vi "UploadImages.vi"(8 "error in (no error)":errorcluster, 11 "Vision in":refnum<class "Vision.lvclass">) -> (0 "error out":errorcluster, 3 "Vision out":refnum<class "Vision.lvclass">)   [LabVIEW 2019, in "Vision.lvlib" / "Vision.lvclass"]
uses:
  Vision.lvclass
  C:/Program Files/National Instruments/LabVIEW 2019/vi.lib/ActorFramework/Actor/Actor.lvclass
  <vilib>/ActorFramework/Actor/Actor.lvclass/Actor.ctl
  Vision.lvclass/Vision.ctl
  Models/ImagesModel.ctl
  Vision Messages/CapturedImage Msg/CapturedImage Msg.lvclass/CapturedImage Msg.ctl
  <vilib>/ActorFramework/Message Enqueuer/Message Enqueuer.lvclass/Message Enqueuer.ctl
  <vilib>/ActorFramework/Message Enqueuer/Enqueue.vi
  Vision Messages/CapturedImage Msg/CapturedImage Msg.lvclass
  C:/Program Files/National Instruments/LabVIEW 2019/vi.lib/ActorFramework/Message/Message.lvclass
  <vilib>/ActorFramework/Message Priority Queue/Priority Enqueue.vi
  <vilib>/ActorFramework/Message Enqueuer/Message Enqueuer.lvclass
  <vilib>/ActorFramework/Actor/Actor.lvclass
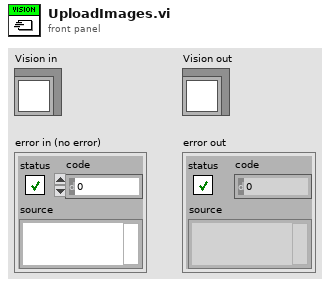
[diagram p1: front panel]
types:
  T1 = typedef "ImagesModel.ctl" = cluster{"guid":string, "images":cluster{"source":string, "rois":string[]}}
  T2 = typedef "IMAQ Image.ctl" = refnum<image>
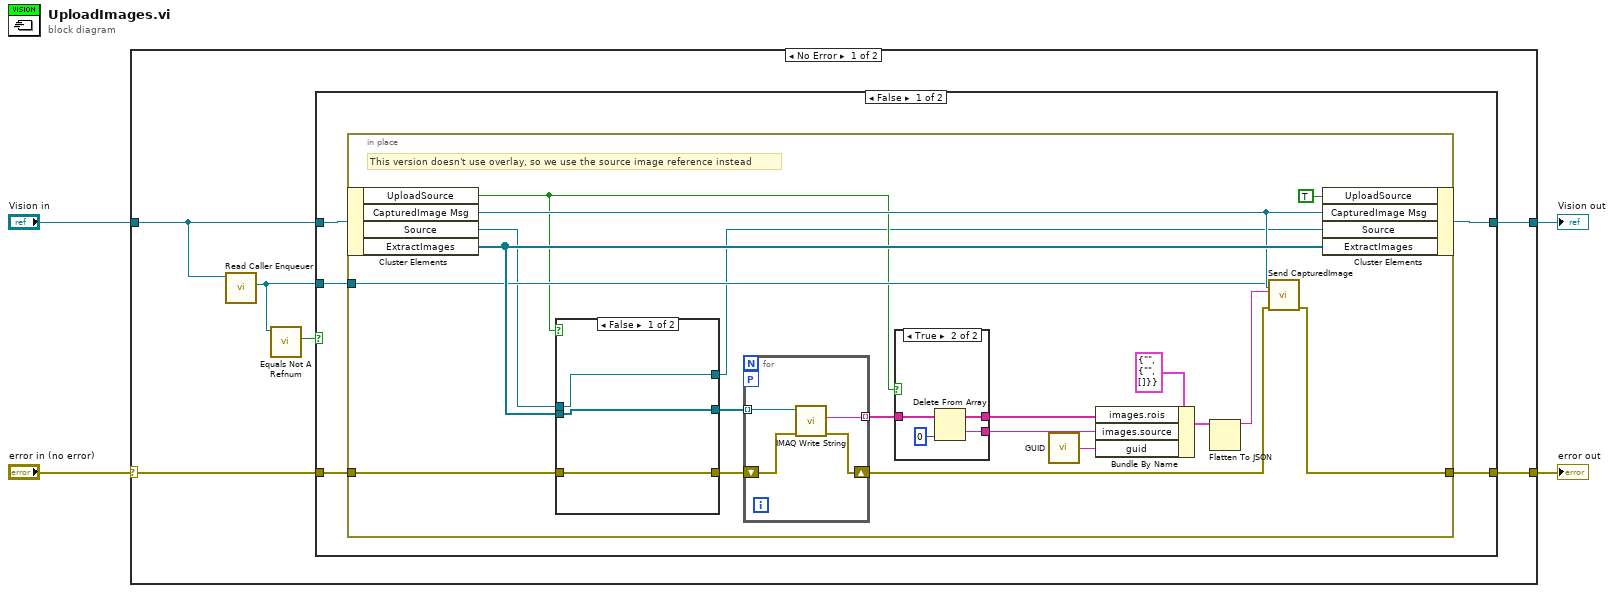
[diagram p0: block diagram]
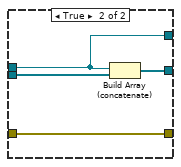
[diagram p2: hidden frame]
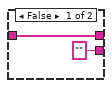
[diagram p3: hidden frame]
diagram:
  n1 = case shown="No Error" "error in (no error)" {
    selector: "error in (no error)" -> [w8 w55]
    tunnel: [w7 w55] -> w3
    tunnel: [w9 w54] -> w1
    tunnel: "Vision in" -> [w10 w54]
    frame No Error {
      n2 = call <vilib>:"Read Caller Enqueuer.vi"("Actor"=w10) -> ("Caller Enqueuer"=w5:refnum<class "Message Enqueuer.lvclass">)  [unwired: 10 in]
      n3 = call <vilib>:"Equals Not A Refnum.vi"("Message Enqueuer"=w5) -> ("Not a refnum?"=w6:bool)  [unwired: 10 in]
      n4 = case shown="False" w6 {
        tunnel: w10 -> [w15 w53]
        tunnel: [w14 w53] -> w9
        tunnel: w8 -> [w13 w52]
        tunnel: [w11 w52] -> w7
        tunnel: w5 -> [w12 _]
        frame False {
          n5 = in-place {
            in-place-border: w13 -> [w19]
            in-place-border: w12 -> [w26]
            in-place-border: [w24] -> w11
            # "This version doesn't use overlay, so we use the source image reference instead"
            n6 = in-place-cluster #1(w15) -> ("UploadSource"=w20:bool, "CapturedImage Msg"=w31:refnum<class "CapturedImage Msg.lvclass">, "Source"=w17:T2, "ExtractImages"=w34:T2[])
            n7 = case shown="False" w20 {
              tunnel: w34 -> [w37 w41]
              tunnel: [w37 w40] -> w33
              tunnel: w19 -> [w36 w38]
              tunnel: [w36 w38] -> w18
              tunnel: [w35 w39] -> w16
              tunnel: w17 -> [w35 w39]
              frame False {
              }
              frame True {
                n8 = Build Array (concatenate)(w39, w41) -> (w40:T2[])
              }
            }
            n9 = for {
              tunnel: w33 -> [w51] mode=indexing
              shift-right: [w49] -> w25
              shift-left: w18 -> [w50]
              tunnel: [w48] -> w32 mode=indexing
              workers-P: _ -> [_]
              n10 = call-poly "IMAQ Write String"("error in (no error)"=w50, "Image"=w51) -> ("error out"=w49:errorcluster, "FileString"=w48:string)  [unwired: 7 in, 1 out]
            }
            n11 = case shown="True" w20 {
              tunnel: w32 -> [w43 w47]
              tunnel: ["" ("FileString") w45] -> w30
              tunnel: [w43 w44] -> w29
              frame False {
              }
              frame True {
                n12 = Delete From Array(array=w47, index=0) -> (deleted portion=w45:string, array with subset deleted=w44:string[])  [unwired: 1 in]
              }
            }
            n13 = call "GUID.vi"() -> ("Guid"=w22:string)  [unwired: 1 in]
            n14 = Bundle By Name(cluster=T1 {"guid"="", "images"={"source"="", "rois"=[]}}, "images.rois"=w29, "images.source"=w30, "guid"=w22) -> (w28:T1)
            n15 = Flatten To JSON(anything=w28) -> (JSON string=w27:string)  [unwired: 2 in, 1 out]
            n16 = call "Send CapturedImage.vi"("Message Type"=w31, "error in (no error)"=w25, "JSON"=w27, "Message Enqueuer"=w26) -> ("error out"=w24:errorcluster)  [unwired: 6 in, 1 out]
            n17 = in-place-cluster #1("UploadSource"=TRUE, "CapturedImage Msg"=w31, "Source"=w16, "ExtractImages"=w34) -> (w14:refnum<class "Vision.lvclass">)
          }
        }
        frame True {
        }
      }
    }
    frame Error {
    }
  }
  "error out" <- w3
  "Vision out" <- w1
